vi "LS 336 T Ramp Act.vi"(0 "command text in":string[](array[string])) -> ()   [LabVIEW 2019]
panel:
  out "Heater Range":enum16{"OFF", "LOW", "MEIDUM", "HIGH"}(ring)
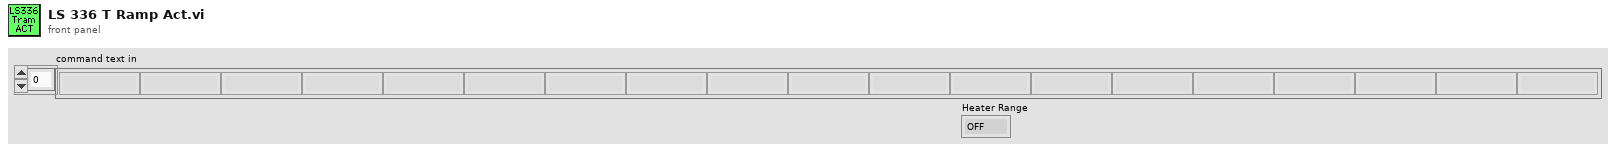
[diagram p1: front panel]
types:
  T1 = typedef "LS 336 T Ramp.ctl" = cluster{"VISA Resource Name":refnum<visa-resource-name>, "extra wait":i32, "start":dbl, "end":dbl, "Sweep Time (H:M:S)":dbl, "Log Linear":bool, "Heater Range":enum16{"OFF", "LOW", "MEIDUM", "HIGH"}, "Loop":bool}
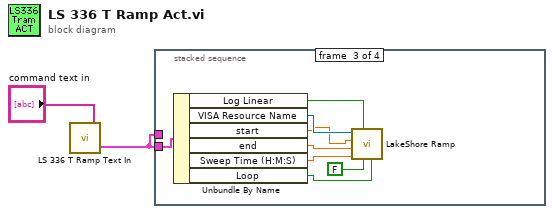
[diagram p0: block diagram]
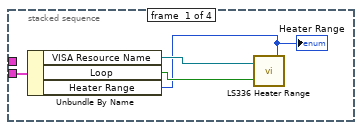
[diagram p2: hidden frame]
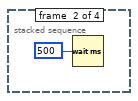
[diagram p3: hidden frame]
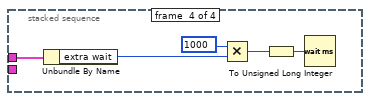
[diagram p4: hidden frame]
diagram:
  n1 = call "LS 336 T Ramp Text In.vi"("command text in"="command text in") -> ("Timed Ramp"=w1:T1)  [unwired: 4 in]
  n2 = stacked-sequence {
    tunnel: w1 -> [w6 _ w15 _]
    tunnel: w1 -> [_ _ _ w17]
    frame #0 {
      n3 = Unbundle By Name(w6) -> ("VISA Resource Name"=w5:refnum<visa-resource-name>, "Loop"=w4:bool, "Heater Range"=w3:enum16{"OFF", "LOW", "MEIDUM", "HIGH"})
      "Heater Range" <- w3
      n4 = call "LS336 Heater Range.vi"("Heater Range"=w3, "Loop"=w4, "Lakeshore GPIB Address"=w5) -> ()
    }
    frame #1 {
      n5 = Wait (ms)(milliseconds to wait=u32 500) -> ()  [unwired: 1 out]
    }
    frame #2 {
      n6 = Unbundle By Name(w15) -> ("Log Linear"=w14:bool, "VISA Resource Name"=w13:refnum<visa-resource-name>, "start"=w12:dbl, "end"=w11:dbl, "Sweep Time (H:M:S)"=w10:dbl, "Loop"=w9:bool)
      n7 = call "LakeShore Ramp.vi"("Loop"=w9, "Parameter"=FALSE, "Mapping"=w14, "Time (Hr:Min:Sec)"=w10, "End Temp/Power"=w11, "Start Temp/Power"=w12, "VISA resource name"=w13) -> ()  [unwired: 5 in]
    }
    frame #3 {
      n8 = Unbundle By Name(w17) -> ("extra wait"=w16:i32)
      n9 = Multiply(x=1000 ("y"), y=w16) -> (x*y=w19:i32)
      n10 = To Unsigned Long Integer(number=w19) -> (unsigned 32bit integer=w18:u32)
      n11 = Wait (ms)(milliseconds to wait=w18) -> ()  [unwired: 1 out]
    }
  }
